vi "Execute.vi"(4 "Iteration":i32, 6 "Time":u32 format="%.3e", 8 "error in (no error)":errorcluster, 9 "Channel Data (DBLs Only)":T4, 10 "Real-Time System Data":T3, 11 "Configuration Data":T2) -> (0 "error out":errorcluster, 1 "Channel Data (DBLs Only)":T4, 2 "Real-Time System Data":T3, 3 "Configuration Data":T2)   [LabVIEW 2014, in "RM interrupt timing Custom Device.lvlib"]
uses:
  RM interrupt timing Custom Device.lvlib
  Real-Time System Data.ctl
  Channel Data.ctl
  Configuration Data.ctl
  <instrlib>/GE 5565 PIORC/GE 5565 PIORC.lvlib
panel:
  out "timeout?":bool
  out "event type":T1(ring)=enum."network interrupt 1"
  out "sender ID":u8
  out "sender data":u32
  # "Controls"
  # "Indicators"
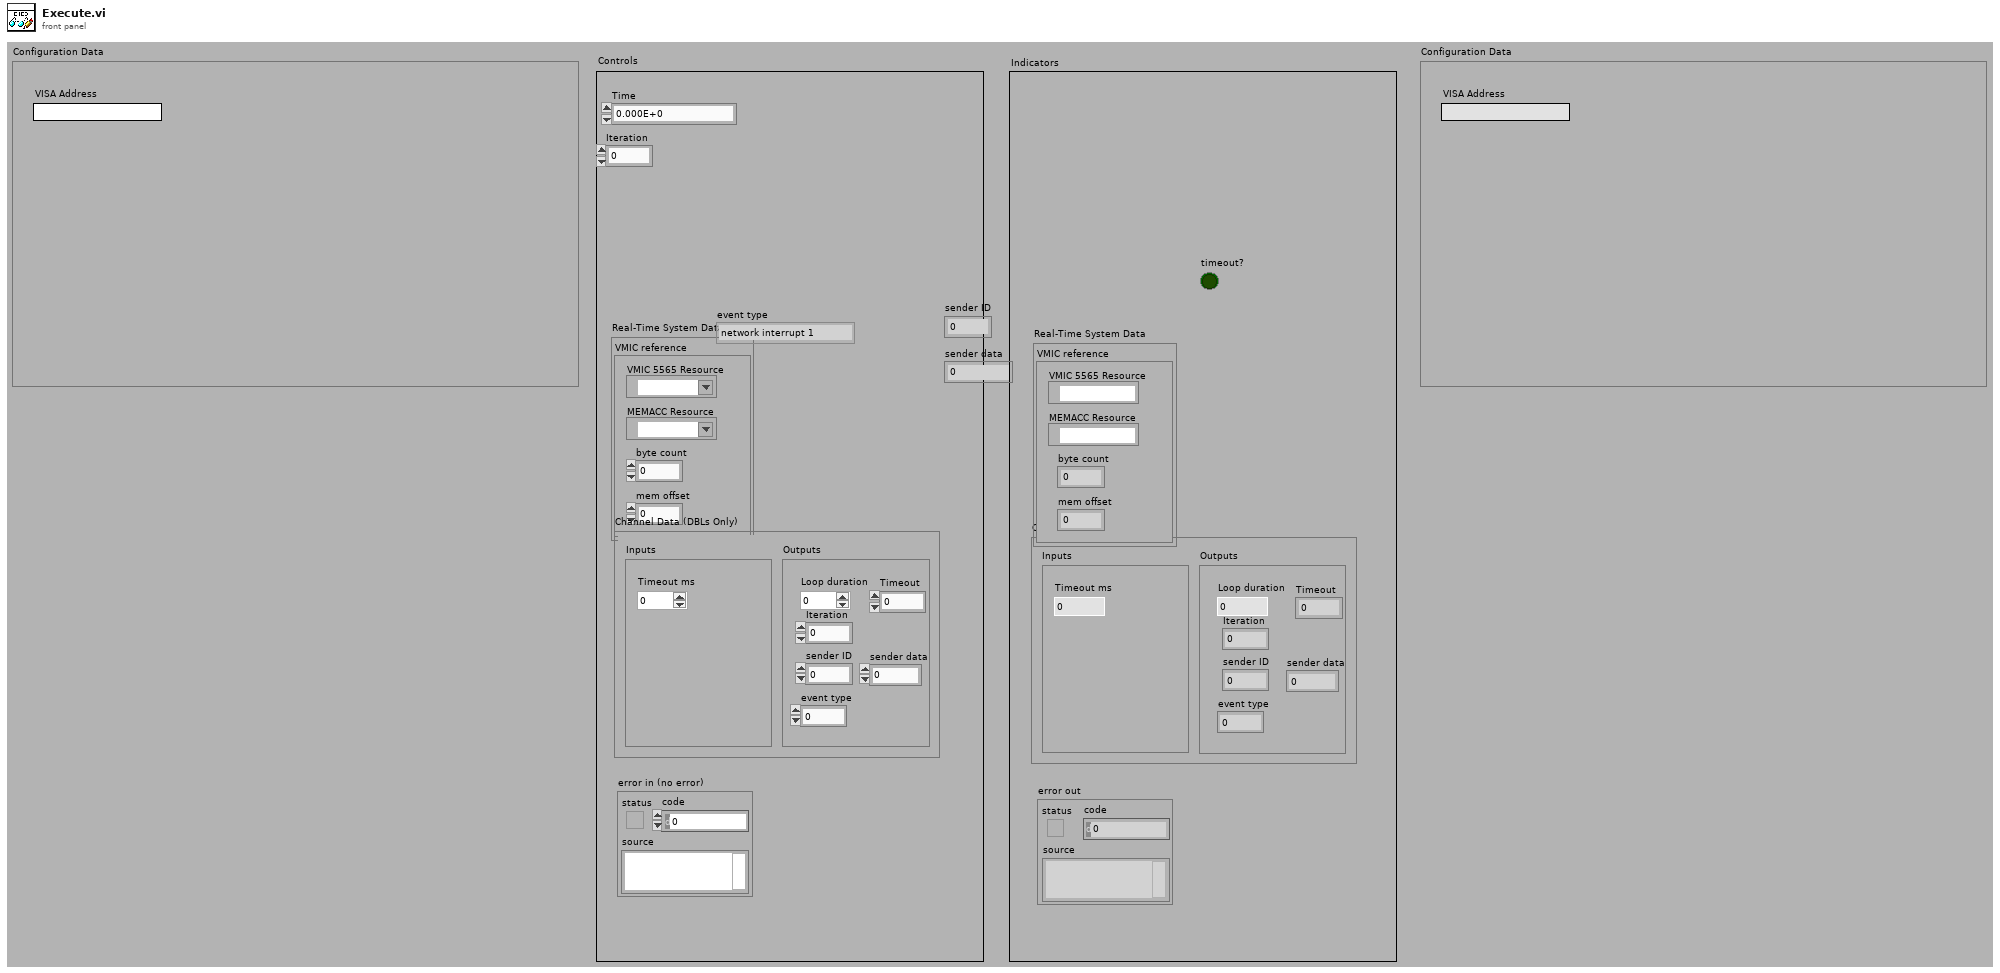
[diagram p1: front panel]
types:
  T1 = enum16{"link reset interrupt", "network interrupt 1", "network interrupt 2", "network interrupt 3", "network init interrupt"}
  T2 = typedef "RM interrupt timing Custom Device.lvlib/Configuration Data.ctl" = cluster{"VISA Address":string}
  T3 = typedef "RM interrupt timing Custom Device.lvlib/Real-Time System Data.ctl" = cluster{"VMIC reference":cluster{"VMIC 5565 Resource":refnum<visa-resource-name>, "MEMACC Resource":refnum<visa-resource-name>, "byte count":u32, "mem offset":u32}}
  T4 = typedef "RM interrupt timing Custom Device.lvlib/Channel Data.ctl" = cluster{"Inputs":cluster{"Timeout ms":dbl}, "Outputs":cluster{"Loop duration":dbl, "Iteration":dbl, "Timeout":dbl, "sender data":dbl, "sender ID":dbl, "event type":dbl}}
  T5 = cluster{"VMIC 5565 Resource":refnum<visa-resource-name>, "MEMACC Resource":refnum<visa-resource-name>, "byte count":u32, "mem offset":u32}
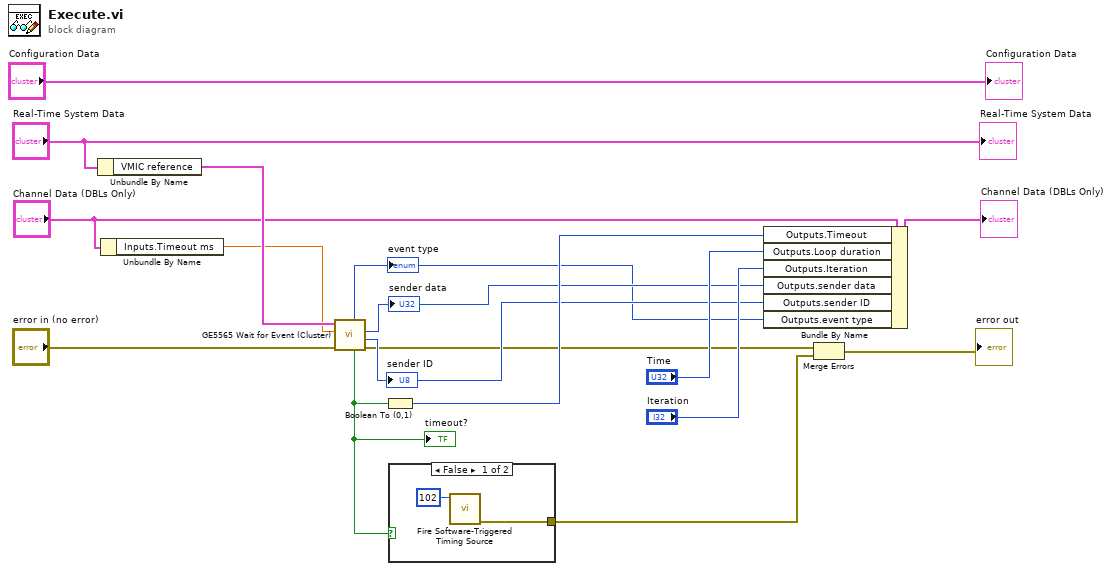
[diagram p0: block diagram]
diagram:
  n1 = Unbundle By Name("Real-Time System Data") -> ("VMIC reference"=w11:T5)
  n2 = Unbundle By Name("Channel Data (DBLs Only)") -> ("Inputs.Timeout ms"=w9:dbl)
  n3 = call <instrlib>:"GE5565 Wait for Event (Cluster).vi"("error in (no error)"="error in (no error)", "timeout (1000 ms)"=w9, "VMIC reference in"=w11) -> ("error out"=w3:errorcluster, "sender ID"=w6:u8, "sender data"=w7:u32, "timeout?"=w4:bool, "event type"=w5:T1)  [unwired: 3 in, 1 out]
  "sender data" <- w7
  "sender ID" <- w6
  "event type" <- w5
  "timeout?" <- w4
  n4 = Boolean To (0,1)(Boolean=w4) -> (0, 1=w8:i16)
  n5 = case shown="False" w4 {
    tunnel: [w18 _] -> w2
    frame False {
      n6 = call <vilib>:"Fire Software-Triggered Timing Source.vi"("trigger ID"=u8 102) -> ("error out"=w18:errorcluster)  [unwired: 9 in, 1 out]
    }
    frame True {
    }
  }
  n7 = Bundle By Name(cluster="Channel Data (DBLs Only)", "Outputs.Timeout"=w8, "Outputs.Loop duration"="Time", "Outputs.Iteration"="Iteration", "Outputs.sender data"=w7, "Outputs.sender ID"=w6, "Outputs.event type"=w5) -> (→"Channel Data (DBLs Only)":T4)
  n8 = Merge Errors(w3, w2) -> (→"error out":errorcluster)
  "Real-Time System Data" <- "Real-Time System Data"
  "Configuration Data" <- "Configuration Data"
